vi "Send Message to Mediator.vi"(8 "error in (no error)":errorcluster caption="错误输入（无错误）", 9 "Message":string, 10 "Receiver":string, 11 "Colleague 输入":refnum<class "Colleague.lvclass"> caption="DNL_LabVIEW Object in") -> (0 "error out":errorcluster caption="错误输出", 3 "Colleague 输出":refnum<class "Colleague.lvclass"> caption="DNL_LabVIEW Object out")   [LabVIEW 2011, in "Colleague.lvclass"]
uses:
  Colleague.lvclass
  Colleague.lvclass/Colleague.ctl
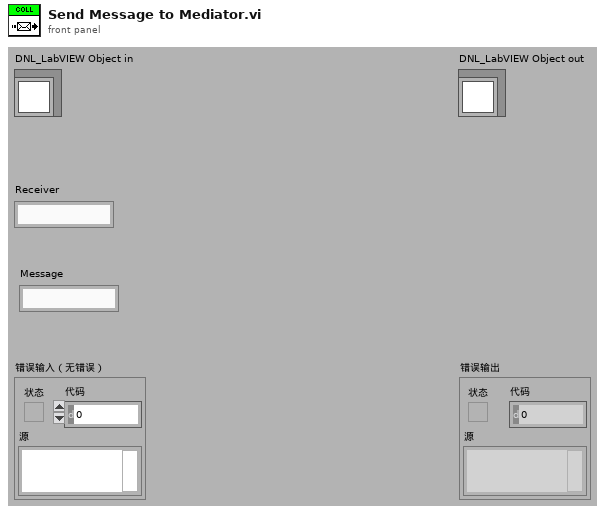
[diagram p1: front panel]
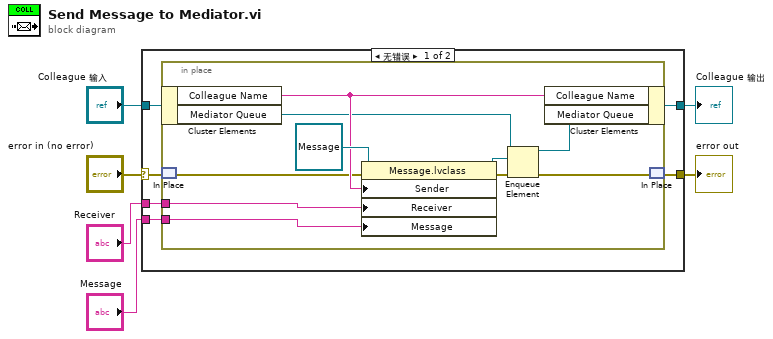
[diagram p0: block diagram]
diagram:
  n1 = case shown="无错误" "error in (no error)" {
    selector: "error in (no error)" -> [w8 w24]
    tunnel: [w7 w24] -> w5
    tunnel: [w9 w23] -> w3
    tunnel: "Colleague 输入" -> [w12 w23]
    tunnel: "Message" -> [w10 _]
    tunnel: "Receiver" -> [w11 _]
    frame No Error {
      n2 = in-place {
        in-place-border: w11 -> [w21]
        in-place-border: w10 -> [w20]
        n3 = in-place-cluster #1(w12) -> ("Colleague Name"=w19:string, "Mediator Queue"=w17:refnum<queue>)
        n4 = in-place-match #2(w8) -> (w18:errorcluster)
        n5 = property class="Message.lvclass"(reference=refnum<class "Message.lvclass"> refnum ("Message.lvclass"), error in=w18, "Sender"=w19, "Receiver"=w21, "Message"=w20) -> (reference out=w15:refnum<class "Message.lvclass">, error out=w14:errorcluster)
        n6 = Enqueue Element(queue=w17, element=w15, error in (no error)=w14) -> (queue out=w16:refnum<queue>, error out=w13:errorcluster)  [unwired: 1 in, 1 out]
        n7 = in-place-cluster #1("Colleague Name"=w19, "Mediator Queue"=w16) -> (w9:refnum<class "Colleague.lvclass">)
        n8 = in-place-match #2(w13) -> (w7:errorcluster)
      }
    }
    frame Error {
    }
  }
  "error out" <- w5
  "Colleague 输出" <- w3
